vi "SubVI_Block Spot #.vi"(5 "Image Register Name":string="untitled", 7 "Magnification":i32 min=0 max=9 step=1, 8 "Error in":errorcluster, 9 "Settings":T4={"Objects"=enum."Bright Objects", "Threshold"=128, "Min Object Size"=FALSE, "Min Size"=3, "Max Object Size"=FALSE, "Max Size"=100} {"Threshold" min=1 max=999999999 step=1; "Max Size" min=1 max=999999999 step=1; "Min Size" min=1 max=999999999 step=1}, 10 "ROI Descriptor":T2 {"Contours"."Type" items=["No Selection", "Point", "Line", "Rectangle", "Oval", "Polygon", "Free", "Annulus", "Unused2", "Unused3", "Broken Line", "Free Hand Line", "Rotated Rectangle"]}, 11 "Image Src In":T1) -> (0 "Error out":errorcluster, 2 "Objects":T3(array[cluster]) {"Area" format="%.2f"; "Object Center"."Y" format="%.2f"; "Object Center"."X" format="%.2f"}, 3 "Image Src Out":T1)   [LabVIEW 2013]
uses:
  <vilib>/vision/Image Controls.llb/IMAQ Image.ctl
  <vilib>/vision/NI_Vision_Development_Module.lvlib
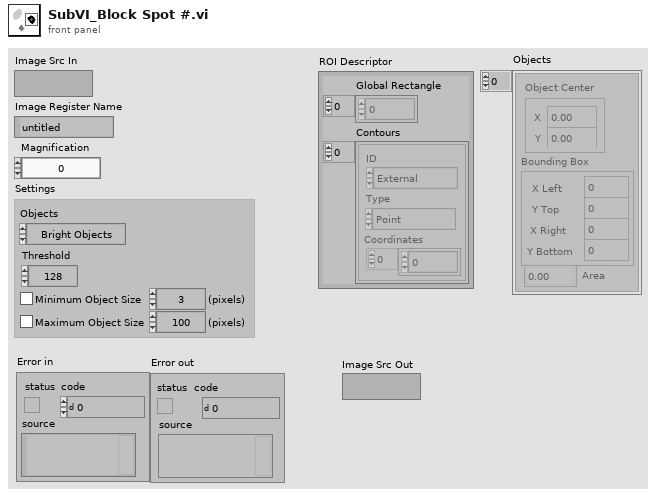
[diagram p1: front panel]
types:
  T1 = typedef "IMAQ Image.ctl" = refnum<image>
  T2 = cluster{"Global Rectangle":i32[], "Contours":cluster{"ID":enum32{"External", "Internal"}, "Type":u32, "Coordinates":i32[]}[]}
  T3 = cluster{"Object Center":cluster{"X":dbl, "Y":dbl}, "Bounding Box":cluster{"X Left":dbl, "Y Top":dbl, "X Right":dbl, "Y Bottom":dbl}, "Area":dbl}[]
  T4 = cluster{"Objects":enum16{"Bright Objects", "Dark Objects"}, "Threshold":i32, "Min Object Size":bool, "Min Size":i32, "Max Object Size":bool, "Max Size":i32}
  T5 = typedef "Particle Parameters" = i32
  T6 = cluster{"Measurement Parameter":T5, "Range Lower Value":dbl, "Range Upper Value":dbl, "Range":bool, "Measurement Type":bool}[]
  T7 = cluster{cluster{dbl, dbl}, cluster{dbl, dbl, dbl, dbl}, dbl}[]
  T8 = typedef "Image Type" = u32
  T9 = cluster{"Measurement Parameter":T5, "Range Lower Value":dbl, "Range Upper Value":dbl, "Range":bool, "Measurement Type":bool}
  T10 = cluster{cluster{dbl, dbl}, cluster{dbl, dbl, dbl, dbl}, dbl}
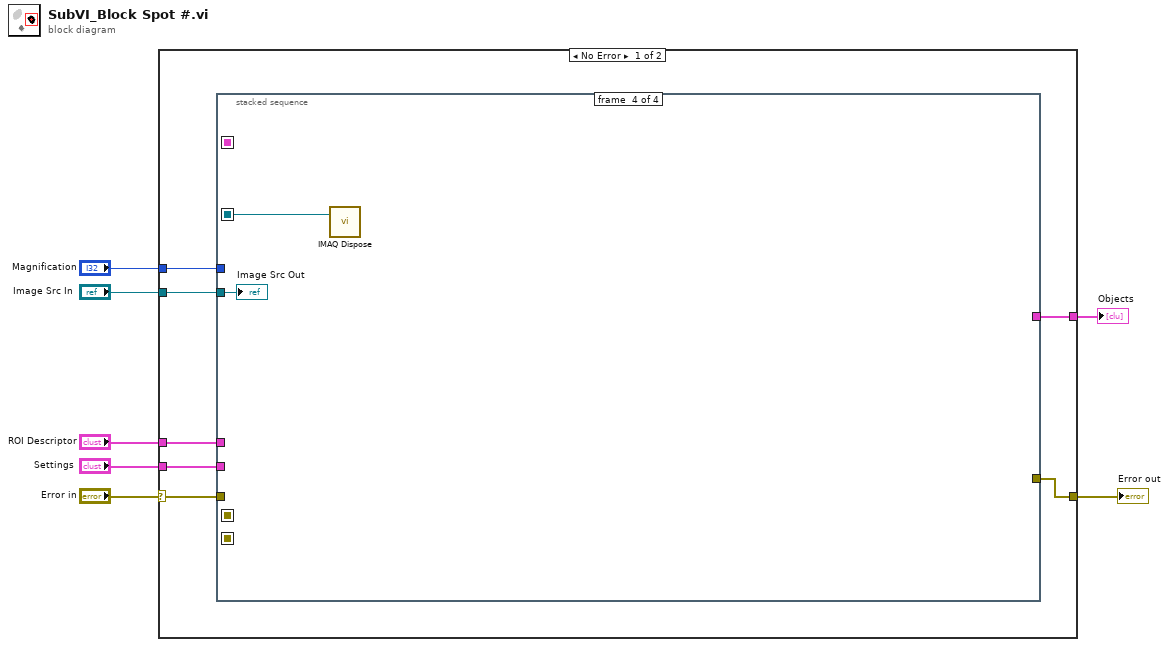
[diagram p0: block diagram]
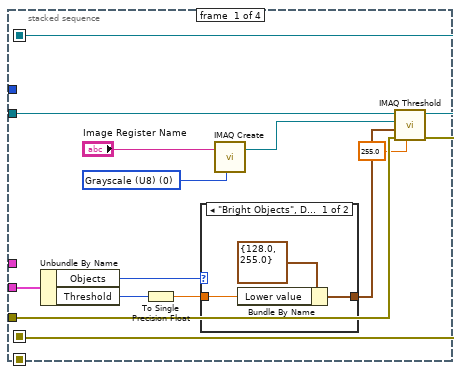
[diagram p2: hidden frame]
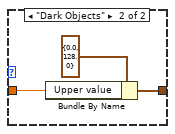
[diagram p3: hidden frame]
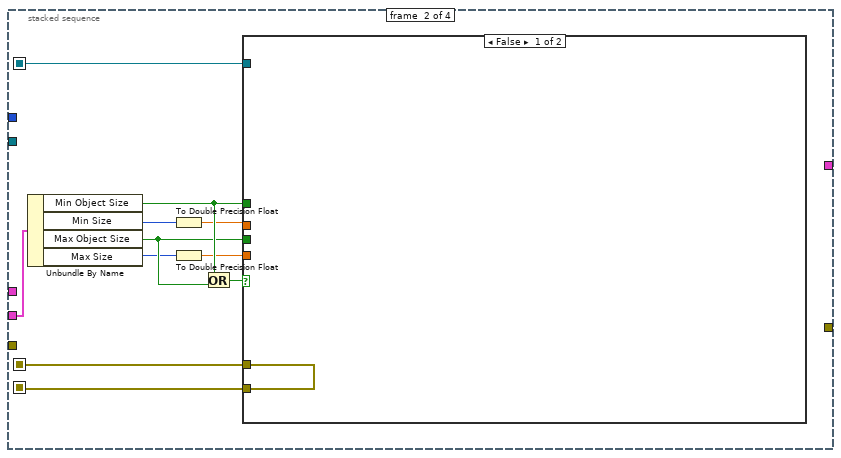
[diagram p4: hidden frame]
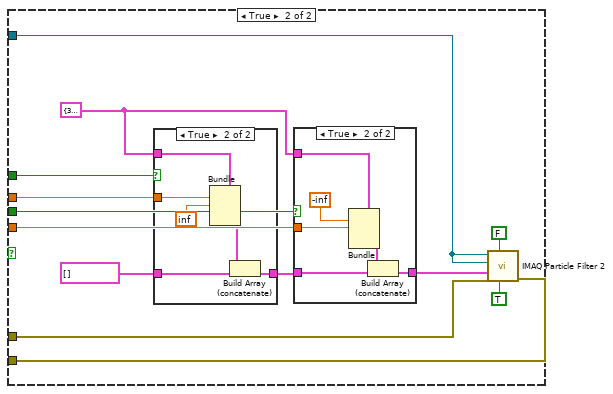
[diagram p5: hidden frame]
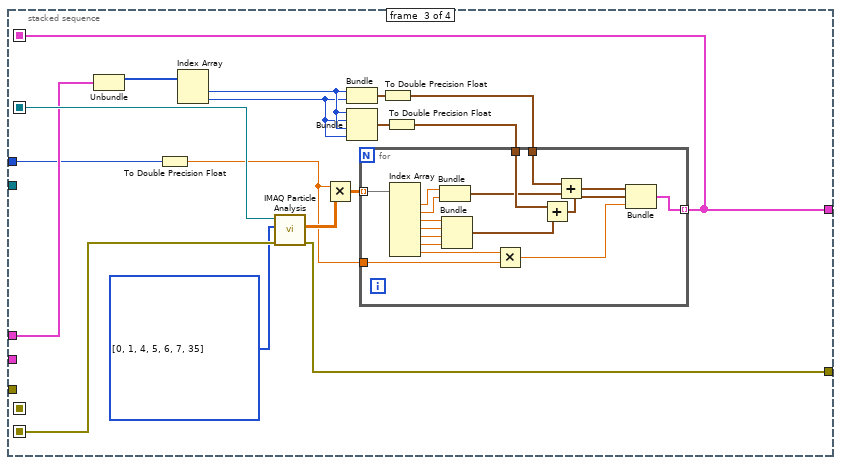
[diagram p8: hidden frame]
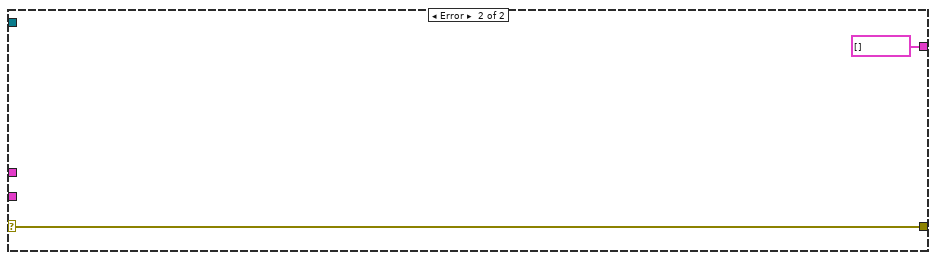
[diagram p9: hidden frame]
diagram:
  n1 = case shown="No Error" "Error in" {
    selector: "Error in" -> [w10 w110]
    tunnel: "Image Src In" -> [w14 _]
    tunnel: "Settings" -> [w13 _]
    tunnel: "ROI Descriptor" -> [w12 _]
    tunnel: "Magnification" -> [w11 _]
    tunnel: [w9 T7 []] -> w2
    tunnel: [w8 w110] -> w1
    frame No Error {
      n2 = stacked-sequence {
        seq-local: [w16 _ _ _] -> [_ w40 w89 w108]
        seq-local: [w17 _ _ _] -> [_ w38 _ _]
        seq-local: [_ _ w74 _] -> [_ _ _ _]
        seq-local: [_ w39 _ _] -> [_ _ w87 _]
        tunnel: w13 -> [w23 w43 _ _]
        tunnel: w14 -> [w24 _ _ w107]
        tunnel: w12 -> [_ _ w88 _]
        tunnel: w10 -> [w27 _ _ _]
        tunnel: w11 -> [_ _ w79 _]
        tunnel: [_ _ w74 _] -> w9
        tunnel: [_ _ w73 _] -> w8
        frame #0 {
          w18 = T8 0 items=["Grayscale (U8)", "Grayscale (I16)", "Grayscale (SGL)", "Complex (CSG)", "RGB (U32)", "HSL (U32)", "RGB (U64)", "Grayscale (U16)"] ("Image Type")
          n3 = Unbundle By Name(w23) -> ("Objects"=w22:enum16{"Bright Objects", "Dark Objects"}, "Threshold"=w21:i32)
          n4 = To Single Precision Float(number=w21) -> (single precision float=w20:sgl)
          n5 = case shown="\"Bright Objects\", Default" w22 {
            tunnel: w20 -> [w30 w32]
            tunnel: [w28 w31] -> w19
            frame "Bright Objects", Default {
              n6 = Bundle By Name(cluster=cluster{"Lower value":sgl, "Upper value":sgl} {"Lower value"=128.0, "Upper value"=255.0} ("Range"), "Lower value"=w30) -> (w28:cluster{"Lower value":sgl, "Upper value":sgl})
            }
            frame "Dark Objects" {
              n7 = Bundle By Name(cluster=cluster{"Lower value":sgl, "Upper value":sgl} {"Lower value"=0.0, "Upper value"=128.0} ("Range"), "Upper value"=w32) -> (w31:cluster{"Lower value":sgl, "Upper value":sgl})
            }
          }
          n8 = call "IMAQ Create"("Image Name"="Image Register Name", "Image Type"=w18) -> ("New Image"=w25:T1)  [unwired: 3 in, 1 out]
          n9 = call "IMAQ Threshold"("Replace Value"=sgl 255.0, "error in (no error)"=w27, "Range"=w19, "Image Dst"=w25, "Image Src"=w24) -> ("error out"=w17:errorcluster, "Image Dst Out"=w16:T1)  [unwired: 1 in, 4 out]
        }
        frame #1 {
          n10 = Unbundle By Name(w43) -> ("Min Object Size"=w42:bool, "Min Size"=w37:i32, "Max Object Size"=w41:bool, "Max Size"=w35:i32)
          n11 = To Double Precision Float(number=w37) -> (double precision float=w36:dbl)
          n12 = To Double Precision Float(number=w35) -> (double precision float=w34:dbl)
          n13 = Or(x=w42, y=w41) -> (x .or. y?=w44:bool)
          n14 = case shown="False" w44 {
            tunnel: w42 -> [_ w58]
            tunnel: w36 -> [_ w57]
            tunnel: w41 -> [_ w56]
            tunnel: w34 -> [_ w55]
            tunnel: w40 -> [_ w46]
            tunnel: w38 -> [w45 w53]
            tunnel: [w45 w52] -> w39
            frame False {
            }
            frame True {
              w50 = T9 {"Measurement Parameter"=35, "Range Lower Value"=0.0, "Range Upper Value"=0.0, "Range"=TRUE, "Measurement Type"=FALSE} ("Selection Value")
              n15 = case shown="True" w58 {
                tunnel: T6 [] ("Selection Values") -> [w66 w72]
                tunnel: w57 -> [_ w69]
                tunnel: [w66 w70] -> w48
                tunnel: w50 -> [_ w67]
                frame False {
                }
                frame True {
                  n16 = Bundle(cluster=w67, "Range Lower Value"=w69, "Range Upper Value"=inf) -> (w71:T9)  [unwired: 3 out]
                  n17 = Build Array (concatenate)(w71, w72) -> (w70:T6)
                }
              }
              n18 = case shown="True" w56 {
                tunnel: w48 -> [w59 w65]
                tunnel: w55 -> [_ w62]
                tunnel: [w59 w63] -> w49
                tunnel: w50 -> [_ w60]
                frame False {
                }
                frame True {
                  n19 = Bundle(cluster=w60, "Range Lower Value"=-inf, "Range Upper Value"=w62) -> (w64:T9)  [unwired: 3 out]
                  n20 = Build Array (concatenate)(w64, w65) -> (w63:T6)
                }
              }
              n21 = call "IMAQ Particle Filter 2"("Keep/Remove Particles (F)"=TRUE ("Keep/Remove Particles"), "Connectivity 4/8 (8)"=FALSE ("Keep/Remove Particles"), "error in (no error)"=w53, "Selection Values"=w49, "Image Dst"=w46, "Image Src"=w46) -> ("error out"=w52:errorcluster)  [unwired: 2 in, 3 out]
            }
          }
        }
        frame #2 {
          w86 = T5[] [0, 1, 4, 5, 6, 7, 35] items=["Center of Mass X", "Center of Mass Y", "First Pixel X", "First Pixel Y", "Bounding Rect Left", "Bounding Rect Top", "Bounding Rect Right", "Bounding Rect Bottom", "Max Feret Diameter Start X", "Max Feret Diameter Start Y", "Max Feret Diameter End X", "Max Feret Diameter End Y", "Max Horiz. Segment Length Left", "Max Horiz. Segment Length Right", "Max Horiz. Segment Length Row", "-", "Bounding Rect Width", "Bounding Rect Height", "Bounding Rect Diagonal", "Perimeter", "Convex Hull Perimeter", "Holes' Perimeter", "Max Feret Diameter", "Equivalent Ellipse Major Axis", "Equivalent Ellipse Minor Axis", "Equivalent Ellipse Minor Axis (Feret)", "Equivalent Rect Long Side", "Equivalent Rect Short Side", "Equivalent Rect Diagonal", "Equivalent Rect Short Side (Feret)", "Average Horiz. Segment Length", "Average Vert. Segment Length", "Hydraulic Radius", "Waddel Disk Diameter", "-", "Area", "Holes' Area", "Particle & Holes' Area", "Convex Hull Area", "Image Area", "-", "Number of Holes", "Number of Horiz. Segments", "Number of Vert. Segments", "-", "Orientation", "Max Feret Diameter Orientation", "-", "% Area/Image Area", "% Area/(Particle & Holes' Area)", "Ratio of Equivalent Ellipse Axes", "Ratio of Equivalent Rect Sides", "-", "Elongation Factor", "Compactness Factor", "Heywood Circularity Factor", "Type Factor", "-", "Sum X", "Sum Y", "Sum XX", "Sum XY", "Sum YY", "Sum XXX", "Sum XXY", "Sum XYY", "Sum YYY", "-", "Moment of Inertia XX", "Moment of Inertia XY", "Moment of Inertia YY", "Moment of Inertia XXX", "Moment of Inertia XXY", "Moment of Inertia XYY", "Moment of Inertia YYY", "Norm. Moment of Inertia XX", "Norm. Moment of Inertia XY", "Norm. Moment of Inertia YY", "Norm. Moment of Inertia XXX", "Norm. Moment of Inertia XXY", "Norm. Moment of Inertia XYY", "Norm. Moment of Inertia YYY", "Hu Moment 1", "Hu Moment 2", "Hu Moment 3", "Hu Moment 4", "Hu Moment 5", "Hu Moment 6", "Hu Moment 7"] ("Pixel Measurements")
          n22 = Unbundle(w88) -> ("Global Rectangle"=w75:i32[])  [unwired: 1 out]
          n23 = To Double Precision Float(number=w79) -> (double precision float=w76:dbl)
          n24 = Index Array(array=w75) -> (element #1=w85:i32, element #2=w84:i32)  [unwired: 2 in]
          n25 = call "IMAQ Particle Analysis"("error in (no error)"=w87, "Pixel Measurements"=w86, "Image"=w89) -> ("error out"=w73:errorcluster, "Particle Measurements (Pixels)"=w78:dbl[][])  [unwired: 2 in, 5 out]
          n26 = Multiply(x=w76, y=w78) -> (x*y=w77:dbl[][])
          n27 = Bundle(w85, w84) -> (w83:cluster{i32, i32})  [unwired: 1 out]
          n28 = Bundle(w85, w84, w85, w84) -> (w81:cluster{i32, i32, i32, i32})  [unwired: 1 out]
          n29 = To Double Precision Float(number=w83) -> (double precision float=w82:cluster{dbl, dbl})
          n30 = To Double Precision Float(number=w81) -> (double precision float=w80:cluster{dbl, dbl, dbl, dbl})
          n31 = for {
            tunnel: w77 -> [w102] mode=indexing
            tunnel: w82 -> [w106]
            tunnel: w80 -> [w105]
            tunnel: [w104] -> w74 mode=indexing
            tunnel: w76 -> [w91]
            n32 = Index Array(array=w102) -> (element #1=w101:dbl, element #2=w100:dbl, element #3=w99:dbl, element #4=w98:dbl, element #5=w97:dbl, element #6=w96:dbl, element #7=w92:dbl)  [unwired: 7 in]
            n33 = Bundle(w101, w100) -> (w94:cluster{dbl, dbl})  [unwired: 1 out]
            n34 = Bundle(w99, w98, w97, w96) -> (w93:cluster{dbl, dbl, dbl, dbl})  [unwired: 1 out]
            n35 = Multiply(x=w92, y=w91) -> (x*y=w90:dbl)
            n36 = Add(x=w105, y=w93) -> (x+y=w103:cluster{dbl, dbl, dbl, dbl})
            n37 = Add(x=w106, y=w94) -> (x+y=w95:cluster{dbl, dbl})
            n38 = Bundle(w95, w103, w90) -> (w104:T10)  [unwired: 1 out]
          }
        }
        frame #3 {
          n39 = call "IMAQ Dispose"("Image"=w108) -> ()  [unwired: 2 in, 4 out]
          "Image Src Out" <- w107
        }
      }
    }
    frame Error {
    }
  }
  "Objects" <- w2
  "Error out" <- w1
